vi "Find and Rename Classes.vi"(0 "Owned Items[]":refnum<vi>[](array[refnum]), 2 "Private Data.Application Ref":refnum<vi>, 5 "New TLB Name":string, 11 "error in":errorcluster) -> (15 "error out":errorcluster)   [LabVIEW 2018, in "Springboard TLB`.lvlib"]
uses:
  Springboard TLB`.lvlib
  <vilib>/regexp/Match Regular Expression.xnode
panel:
  out "Array 2":string[](array[string])
  out "Array":string[](array[string])
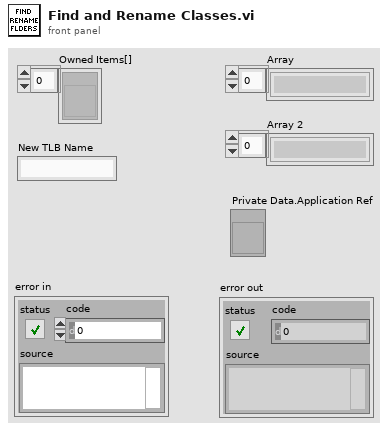
[diagram p1: front panel]
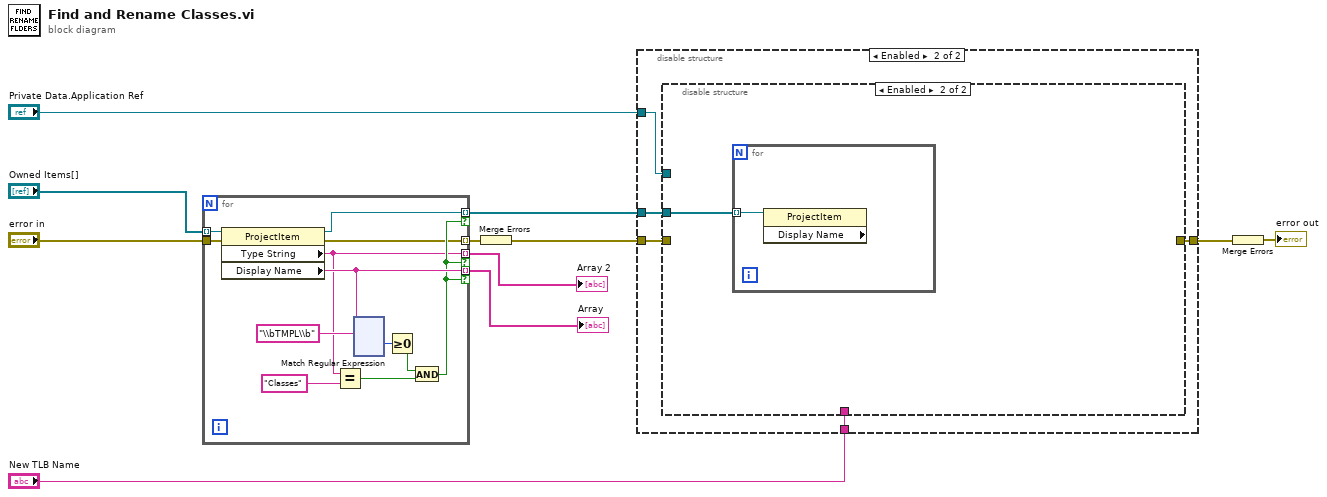
[diagram p0: block diagram]
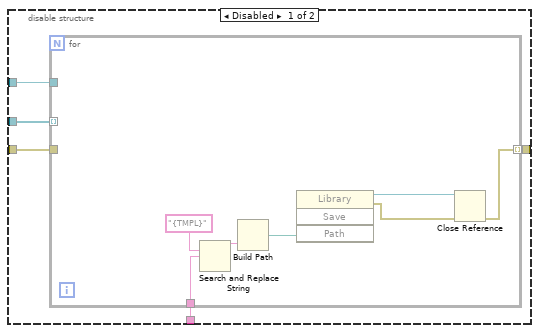
[diagram p3: hidden frame]
diagram:
  n1 = for {
    tunnel: "Owned Items[]" -> [w23] mode=indexing
    tunnel: [w14] -> w6 mode=indexing if=w18
    tunnel: [w21] -> w7 mode=indexing if=w18
    tunnel: [w12] -> w1 mode=indexing if=w18
    tunnel: [w17] -> w10 mode=indexing
    tunnel: "error in" -> [w16]
    n2 = property class="ProjectItem"(reference=w23, error in=w16) -> (reference out=w12:refnum<vi>, error out=w17:errorcluster, "Type String"=w14:string, "Display Name"=w21:string)
    n3 = Equal?(x=w14, y="Classes") -> (x = y?=w13:bool)
    n4 = xnode "Match Regular Expression"("input string"=w21, "regular expression"="\\bTMPL\\b") -> ("offset past match"=w19:i32)  [unwired: 4 in, 4 out]
    n5 = Greater Or Equal To 0?(x=w19) -> (x >= 0?=w15:bool)
    n6 = And(x=w15, y=w13) -> (x .and. y?=w18:bool)
  }
  "Array" <- w7
  "Array 2" <- w6
  n7 = Merge Errors(w10) -> (w11:errorcluster)
  n8 = disable-structure shown="Enabled" {
    disable-tunnel: w11 -> [w138 w141]
    disable-tunnel: "New TLB Name" -> [_ w139]
    disable-tunnel: [w138 w140] -> w4
    disable-tunnel: "Private Data.Application Ref" -> [_ w143]
    disable-tunnel: w1 -> [_ w142]
    frame Disabled {
    }
    frame Enabled {
      n9 = disable-structure shown="Enabled" {
        disable-tunnel: w143 -> [w148 _]
        disable-tunnel: w142 -> [w147 w160]
        disable-tunnel: w141 -> [w146 _]
        disable-tunnel: [w145 _] -> w140
        disable-tunnel: w139 -> [w144 _]
        frame Disabled {
          n10 = for {
            tunnel: w148 -> [_]
            tunnel: w147 -> [_] mode=indexing
            tunnel: w146 -> [_]
            tunnel: [w155] -> w145 mode=indexing
            tunnel: w144 -> [w150]
            n11 = Search and Replace String(search string="{TMPL}", replace string=w150) -> (input string=w154:string, result string=w152:string)  [unwired: 5 in, 3 out]
            n12 = Build Path(name or relative path=w152) -> (base path=w151:path, appended path=w149:path)
            n13 = invoke class="Library" method="Save"("Path"=w149) -> (reference=w159:refnum<vi>, reference out=w156:refnum<vi>, error in=w158:errorcluster, error out=w157:errorcluster)  [unwired: 1 in, 2 out]
            n14 = Close Reference(reference=w156, error in (no error)=w157) -> (error out=w155:errorcluster)
          }
        }
        frame Enabled {
          n15 = for {
            tunnel: w160 -> [w161] mode=indexing
            n16 = property class="ProjectItem" props=["Display Name"](reference=w161) -> ()  [unwired: 1 in, 3 out]
          }
        }
      }
    }
  }
  n17 = Merge Errors(w4) -> (→"error out":errorcluster)
